vi "Swap Channels.vi"(7 "Wfm Data":waveform(sgl)[](array[waveform])) -> (8 "Wfm Data out":waveform(sgl)[](array[waveform]))   [LabVIEW 2014]
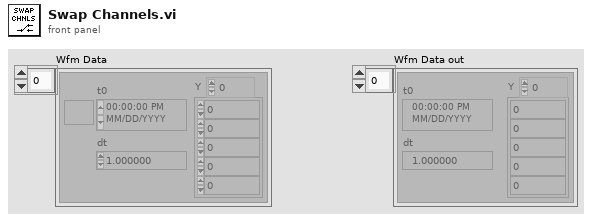
[diagram p1: front panel]
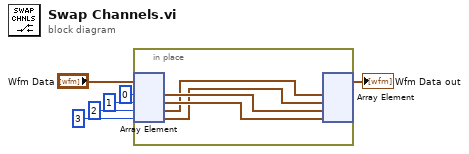
[diagram p0: block diagram]
diagram:
  n1 = in-place {
    n2 = in-place-array #1("Wfm Data", 0, 1, 2, 3) -> (w10:waveform(sgl), w9:waveform(sgl), w8:waveform(sgl), w7:waveform(sgl))
    n3 = in-place-array #1(w8, w7, w10, w9) -> (→"Wfm Data out":waveform(sgl)[])  [unwired: 4 out]
  }
